vi "Process.vi"(8 "error in":errorcluster, 11 "Plugin in":refnum<class "FFT.lvclass">) -> (0 "error out":errorcluster, 3 "Plugin out":refnum<class "FFT.lvclass">)   [LabVIEW 2024, in "FFT.lvlib" / "FFT.lvclass"]
uses:
  FFT.lvclass
  C:/Program Files/National Instruments/LabVIEW 2024/vi.lib/FlexLogger/SDK/PluginSDK.lvlibp/PEFClasses/SDK/Plugin/Plugin.lvclass
  FFT.lvclass/FFT.ctl
  <vilib>/Analysis/2dsp.llb/Power Spectrum (DBL).vi
  <vilib>/FlexLogger/SDK/PluginSDK.lvlibp/PEFClasses/SDK/Plugin/DataHelpers/Write 1D Wfm (DBL)_v2.vi
  <vilib>/FlexLogger/SDK/PluginSDK.lvlibp/PEFClasses/SDK/Plugin/Plugin.lvclass
  <vilib>/Analysis/NI_AALPro.lvlib
  C:/Program Files/National Instruments/LabVIEW 2024/vi.lib/FlexLogger/SDK/PluginSDK.lvlibp/PEFClasses/SDK/Processing Element/Processing Element.lvclass
  C:/dev/niflexlogger-plugins/plugins/FFT/source/FFT.lvclass
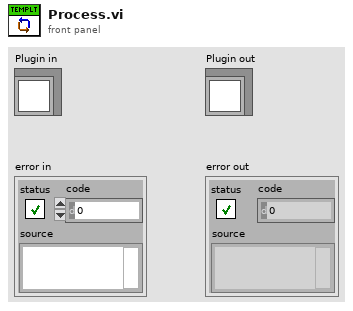
[diagram p1: front panel]
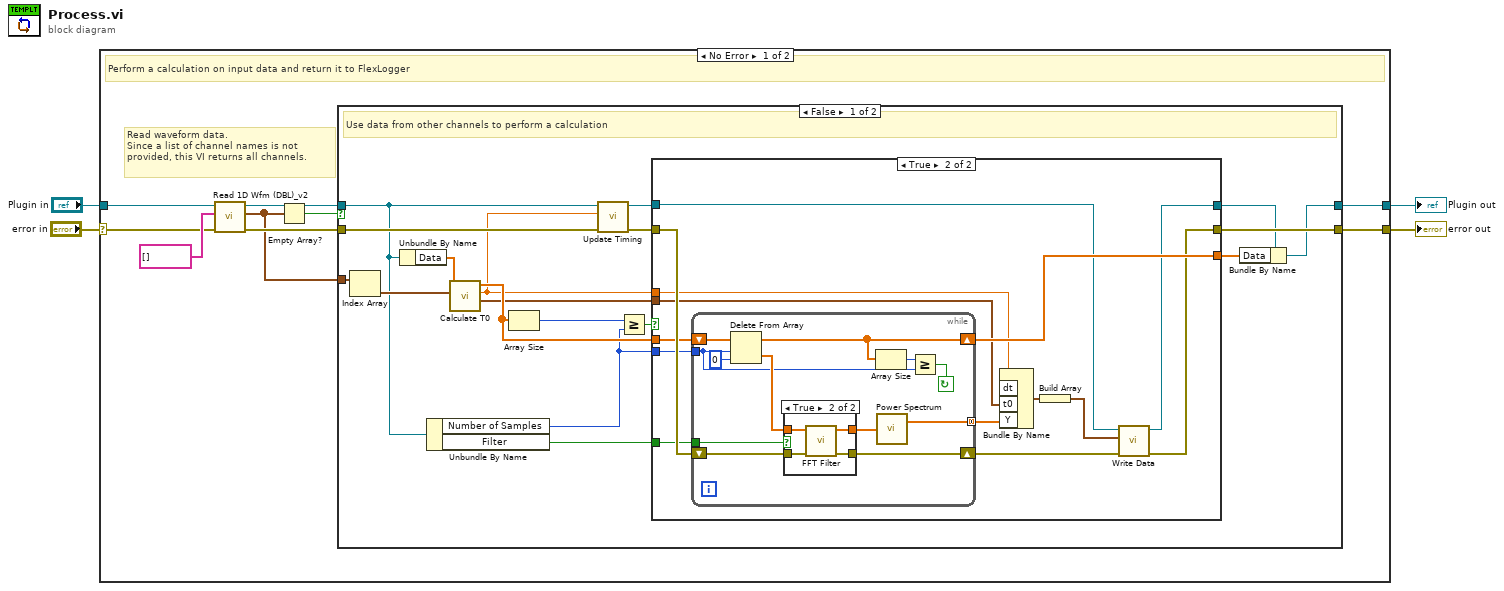
[diagram p0: block diagram]
diagram:
  n1 = case shown="No Error" "error in" {
    selector: "error in" -> [w7 w69]
    tunnel: [w12 w70] -> w1
    tunnel: "Plugin in" -> [w5 w70]
    tunnel: [w13 w69] -> w2
    frame No Error {
      # "Read waveform data.\nSince a list of channel names is not provided, this VI returns all channels."
      # "Perform a calculation on input data and return it to FlexLogger"
      n2 = call <vilib>:"Read 1D Wfm (DBL)_v2.vi"("error in (no error)"=w7, "Unique Identifers (empty = all)"=string[] [] ("Unique Channel Identifers (empty = all)"), "Plugin in"=w5) -> ("error out"=w11:errorcluster, "Data"=w8:waveform(dbl)[], "Plugin out"=w9:refnum<class "FFT.lvclass">)  [unwired: 5 in, 1 out]
      n3 = Empty Array?(array=w8) -> (empty?=w6:bool)
      n4 = case shown="False" w6 {
        tunnel: [w31 w67] -> w13
        tunnel: [w23 w68] -> w12
        tunnel: w9 -> [w16 w68]
        tunnel: w11 -> [w21 w67]
        tunnel: w8 -> [w30 _]
        frame False {
          # "Use data from other channels to perform a calculation"
          n5 = Index Array(array=w30) -> (element=w29:waveform(dbl))  [unwired: 1 in]
          n6 = Unbundle By Name(w16) -> ("Data"=w28:dbl[])
          n7 = Unbundle By Name(w16) -> ("Number of Samples"=w15:i32, "Filter"=w14:bool)
          n8 = call "Calculate T0.vi"("Waveform"=w29, "Data In"=w28) -> ("Data Out T0"=w18:timestamp, "dt"=w17:dbl, "Data Out"=w19:dbl[])  [unwired: 7 in]
          n9 = Array Size(array=w19) -> (size(s)=w27:i32)
          n10 = call "Update Timing.vi"("error in (no error)"=w21, "dt(sec)"=w17, "FFT Ref In"=w16) -> ("error out"=w20:errorcluster, "FFT Ref Out"=w22:refnum<class "FFT.lvclass">)  [unwired: 7 in]
          n11 = Greater Or Equal?(x=w27, y=w15) -> (x >= y?=w26:bool)
          n12 = case shown="True" w26 {
            tunnel: [w34 w43] -> w31
            tunnel: [w33 w36] -> w25
            tunnel: w20 -> [w34 w47]
            tunnel: w22 -> [w33 w37]
            tunnel: w19 -> [w32 w46]
            tunnel: w15 -> [_ w45]
            tunnel: [w32 w44] -> w24
            tunnel: w18 -> [_ w41]
            tunnel: w17 -> [_ w40]
            tunnel: w14 -> [_ w35]
            frame False {
            }
            frame True {
              n13 = while {
                tunnel: w45 -> [w49]
                shift-right: [w59] -> w48
                shift-left: w47 -> [w51]
                shift-right: [w55] -> w44
                shift-left: w46 -> [w58]
                tunnel: [w54] -> w42 mode=concatenating
                tunnel: w35 -> [w50]
                stop <- w52 continue-if-true
                n14 = Delete From Array(array=w58, length=w49, index=0) -> (deleted portion=w56:dbl[], array with subset deleted=w55:dbl[])
                n15 = case shown="True" w50 {
                  tunnel: [w61 w65] -> w60
                  tunnel: w51 -> [w62 w66]
                  tunnel: [w62 w64] -> w59
                  tunnel: w56 -> [w61 w63]
                  frame False {
                  }
                  frame True {
                    n16 = call "FFT Filter.vi"("error in"=w66, "Data in"=w63) -> ("error out"=w64:errorcluster, "Data out"=w65:dbl[])  [unwired: 8 in]
                  }
                }
                n17 = Array Size(array=w55) -> (size(s)=w53:i32)
                n18 = call-poly <vilib>:"Power Spectrum.vi"("X"=w60) -> ("Power Spectrum"=w54:dbl[])  [unwired: 1 out]
                n19 = Greater Or Equal?(x=w53, y=w49) -> (x >= y?=w52:bool)
              }
              n20 = Bundle By Name("dt"=w40, "t0"=w41, "Y"=w42) -> (w39:waveform(dbl))  [unwired: 1 in]
              n21 = Build Array(w39) -> (w38:waveform(dbl)[])
              n22 = call-poly <vilib>:"Write Data.vi"("error in (no error)"=w48, "Data"=w38, "Plugin in"=w37) -> ("error out"=w43:errorcluster, "Plugin out"=w36:refnum<class "FFT.lvclass">)  [unwired: 7 in]
            }
          }
          n23 = Bundle By Name(cluster=w25, "Data"=w24) -> (w23:refnum<class "FFT.lvclass">)
        }
        frame True {
          # "No channels sending data to the plugin"
        }
      }
    }
    frame Error {
    }
  }
  "error out" <- w2
  "Plugin out" <- w1
